vi "Test output clocks.vi"() -> ()   [LabVIEW 2020]
uses:
  <vilib>/DAQmx/write.llb/DAQmx Write (Analog 1D DBL 1Chan NSamp).vi
  <vilib>/DAQmx/create/channels.llb/DAQmx Create Channel (AO-Voltage-Basic).vi
  <vilib>/DAQmx/create/channels.llb/DAQmx Create Channel (CO-Pulse Generation-Frequency).vi
  <vilib>/DAQmx/configure/timing.llb/DAQmx Timing (Implicit).vi
  <vilib>/DAQmx/configure/timing.llb/DAQmx Timing (Sample Clock).vi
  <vilib>/DAQmx/miscellaneous.llb/DAQmx Fill In Error Info.vi
  <vilib>/DAQmx/create/channels.llb/DAQmx Create Channel (CO-Pulse Generation-Ticks).vi
  <resource>/objmgr/daqmx.rc
panel:
  out "AI CO.Pulse.Freq":dbl
  in  "AI counter":tag="6251/ctr1"
  in  "AI rate divider":i32
  out "SampTimingType":i32(ring)=10451 items=["Sample Clock"=10388, "Burst Handshake"=12548, "Handshake"=10389, "Implicit"=10451, "On Demand"=10390, "Change Detection"=12504, "Pipelined Sample Clock"=14668]
  out "CO SampClk.Rate":dbl=3809523.8095238097
  in  "AO counter":tag="6251/ctr0"
  out "AO SampClk.Rate":dbl=3809523.8095238097 format="%#.8p"
  in  "data":dbl[](array[numeric])=[0.0, 1.0, 0.0] format="%0.2f"
  in  "AO rate":dbl=3800000.0 format="%.4p"
  in  "Output channels":tag="6251/ao0"
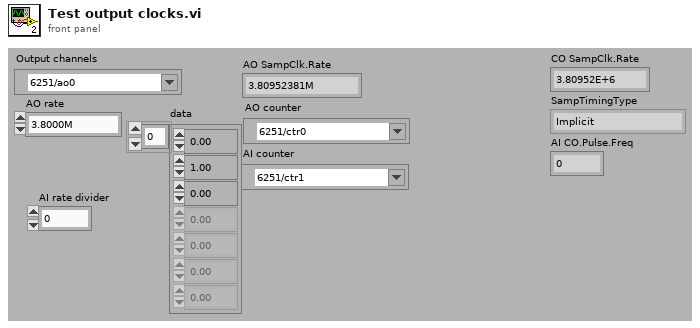
[diagram p1: front panel]
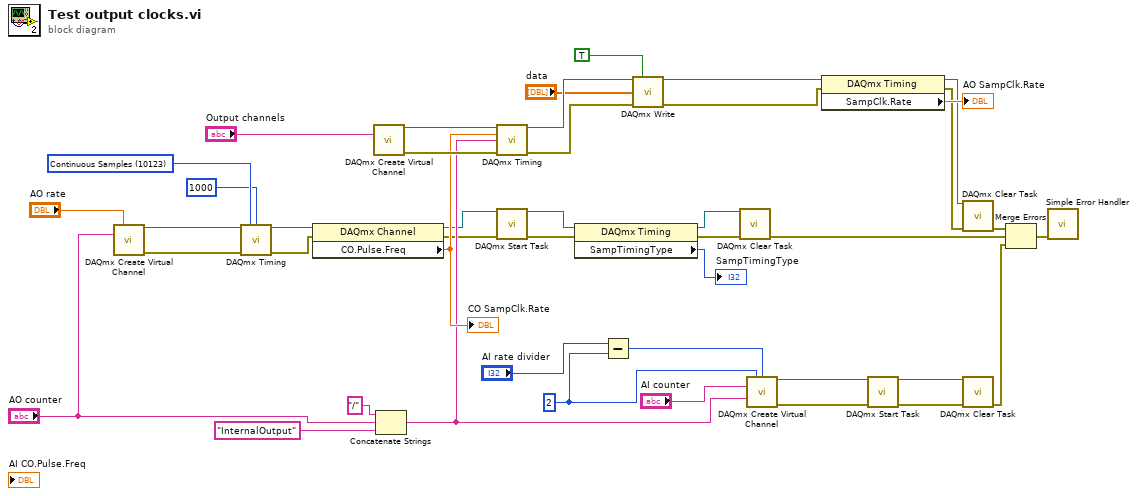
[diagram p0: block diagram]
diagram:
  w17 = u32 2 ("high ticks")
  w25 = 10123 items=["Finite Samples"=10178, "Continuous Samples"=10123, "Hardware Timed Single Point"=12522] ("sample mode")
  n1 = call-poly <vilib>:"DAQmx Create Virtual Channel.vi"("frequency"="AO rate", "counter"="AO counter") -> ("task out"=w31:refnum<k21>, "error out"=w30:errorcluster)  [unwired: 12 in]
  n2 = call-poly <vilib>:"DAQmx Timing.vi"("task/channels in"=w31, "sample mode"=w25, "samples per channel"=1000, "error in"=w30) -> ("task out"=w6:refnum<k21>, "error out"=w8:errorcluster)  [unwired: 10 in]
  n3 = property class="DAQmx Channel"(reference=w6, error in=w8) -> (reference out=w5:refnum<k21>, error out=w7:errorcluster, "CO.Pulse.Freq"=w18:dbl)
  "CO SampClk.Rate" <- w18
  n4 = call-poly <vilib>:"DAQmx Create Virtual Channel.vi"("physical channels"="Output channels") -> ("task out"=w40:refnum<k21>, "error out"=w39:errorcluster)  [unwired: 13 in]
  n5 = Concatenate Strings("/", "AO counter", "InternalOutput" ("string")) -> (w14:string)
  n6 = call-poly <vilib>:"DAQmx Timing.vi"("task/channels in"=w40, "rate"=w18, "source"=w14, "error in"=w39) -> ("task out"=w42:refnum<k21>, "error out"=w41:errorcluster)  [unwired: 10 in]
  n7 = call <vilib>:"DAQmx Start Task.vi"("task/channels in"=w5, "error in"=w7) -> ("task out"=w23:refnum<k21>, "error out"=w29:errorcluster)  [unwired: 12 in]
  n8 = property class="DAQmx Timing"(reference=w23, error in=w29) -> (reference out=w27:refnum<k21>, error out=w28:errorcluster, "SampTimingType"=→"SampTimingType":i32)
  n9 = Subtract(x="AI rate divider", y=w17) -> (x-y=w16:u32)
  n10 = call-poly <vilib>:"DAQmx Write.vi"("task/channels in"=w42, "auto start"=TRUE, "data"="data", "error in"=w41) -> ("task out"=w37:refnum<k21>, "error out"=w36:errorcluster)  [unwired: 9 in, 1 out]
  n11 = call <vilib>:"DAQmx Clear Task.vi"("task in"=w27, "error in"=w28) -> ("error out"=w3:errorcluster)  [unwired: 13 in]
  n12 = call-poly <vilib>:"DAQmx Create Virtual Channel.vi"("high ticks"=w17, "low ticks"=w16, "counter"="AI counter", "source of ticks"=w14) -> ("task out"=w11:refnum<k21>, "error out"=w12:errorcluster)  [unwired: 5 in, 5 out]
  n13 = property class="DAQmx Timing"(reference=w37, error in=w36) -> (reference out=w32:refnum<k21>, error out=w33:errorcluster, "SampClk.Rate"=→"AO SampClk.Rate":dbl)
  n14 = call <vilib>:"DAQmx Start Task.vi"("task/channels in"=w11, "error in"=w12) -> ("task out"=w9:refnum<k21>, "error out"=w10:errorcluster)  [unwired: 12 in]
  n15 = call <vilib>:"DAQmx Clear Task.vi"("task in"=w32, "error in"=w33) -> ("error out"=w4:errorcluster)  [unwired: 13 in]
  n16 = call <vilib>:"DAQmx Clear Task.vi"("task in"=w9, "error in"=w10) -> ("error out"=w2:errorcluster)  [unwired: 13 in]
  n17 = Merge Errors(w4, w3, w2) -> (w1:errorcluster)
  n18 = call <vilib>:"Simple Error Handler.vi"("error in (no error)"=w1) -> ()  [unwired: 4 in, 5 out]
